vi "PKYK_Result_String.vi"(11 "Result":T1) -> (1 "color(black) 2":u32, 2 "color(black)":u32, 3 "RFID Written Last":string)   [LabVIEW 2020]
uses:
  Controls/PKYK_Status.ctl
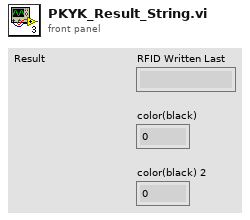
[diagram p1: front panel]
types:
  T1 = typedef "PKYK_Status.ctl" = u16
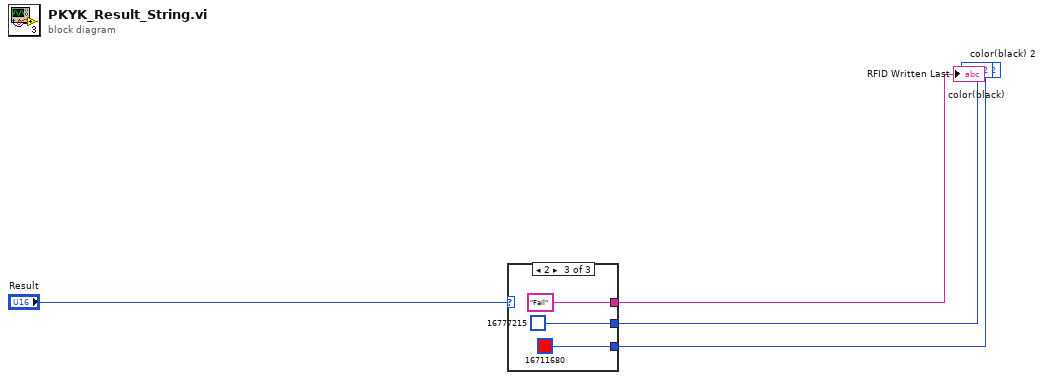
[diagram p0: block diagram]
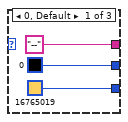
[diagram p2: hidden frame]
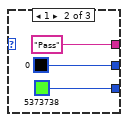
[diagram p3: hidden frame]
diagram:
  n1 = case shown="2" "Result" {
    tunnel: ["--" ("RFID Written Last") "Pass" ("RFID Written Last") "Fail" ("RFID Written Last")] -> w3
    tunnel: [u32 0 ("color(black)") u32 0 ("color(black)") u32 16777215 ("color(black)")] -> w2
    tunnel: [u32 16765019 ("color(black)") u32 5373738 ("color(black)") u32 16711680 ("color(black)")] -> w1
    frame 0, Default {
    }
    frame 1 {
    }
    frame 2 {
    }
  }
  "RFID Written Last" <- w3
  "color(black)" <- w2
  "color(black) 2" <- w1
